vi "ImageCapture.vi"() -> ()   [LabVIEW 2021]
uses:
  <vilib>/userdefined/High Color/IMAQdx.ctl
  <vilib>/vision/driver/NI_Vision_Acquisition_Software.lvlib
panel:
  out "path":path
  out "error out 3":errorcluster
  in  "Ref":path
  in  "Snap?":bool
  out "error out 2":errorcluster
  out "error out":errorcluster
  out "Image":T1(plugin-control)
  in  "Camera Source":T2
  in  "stop":bool
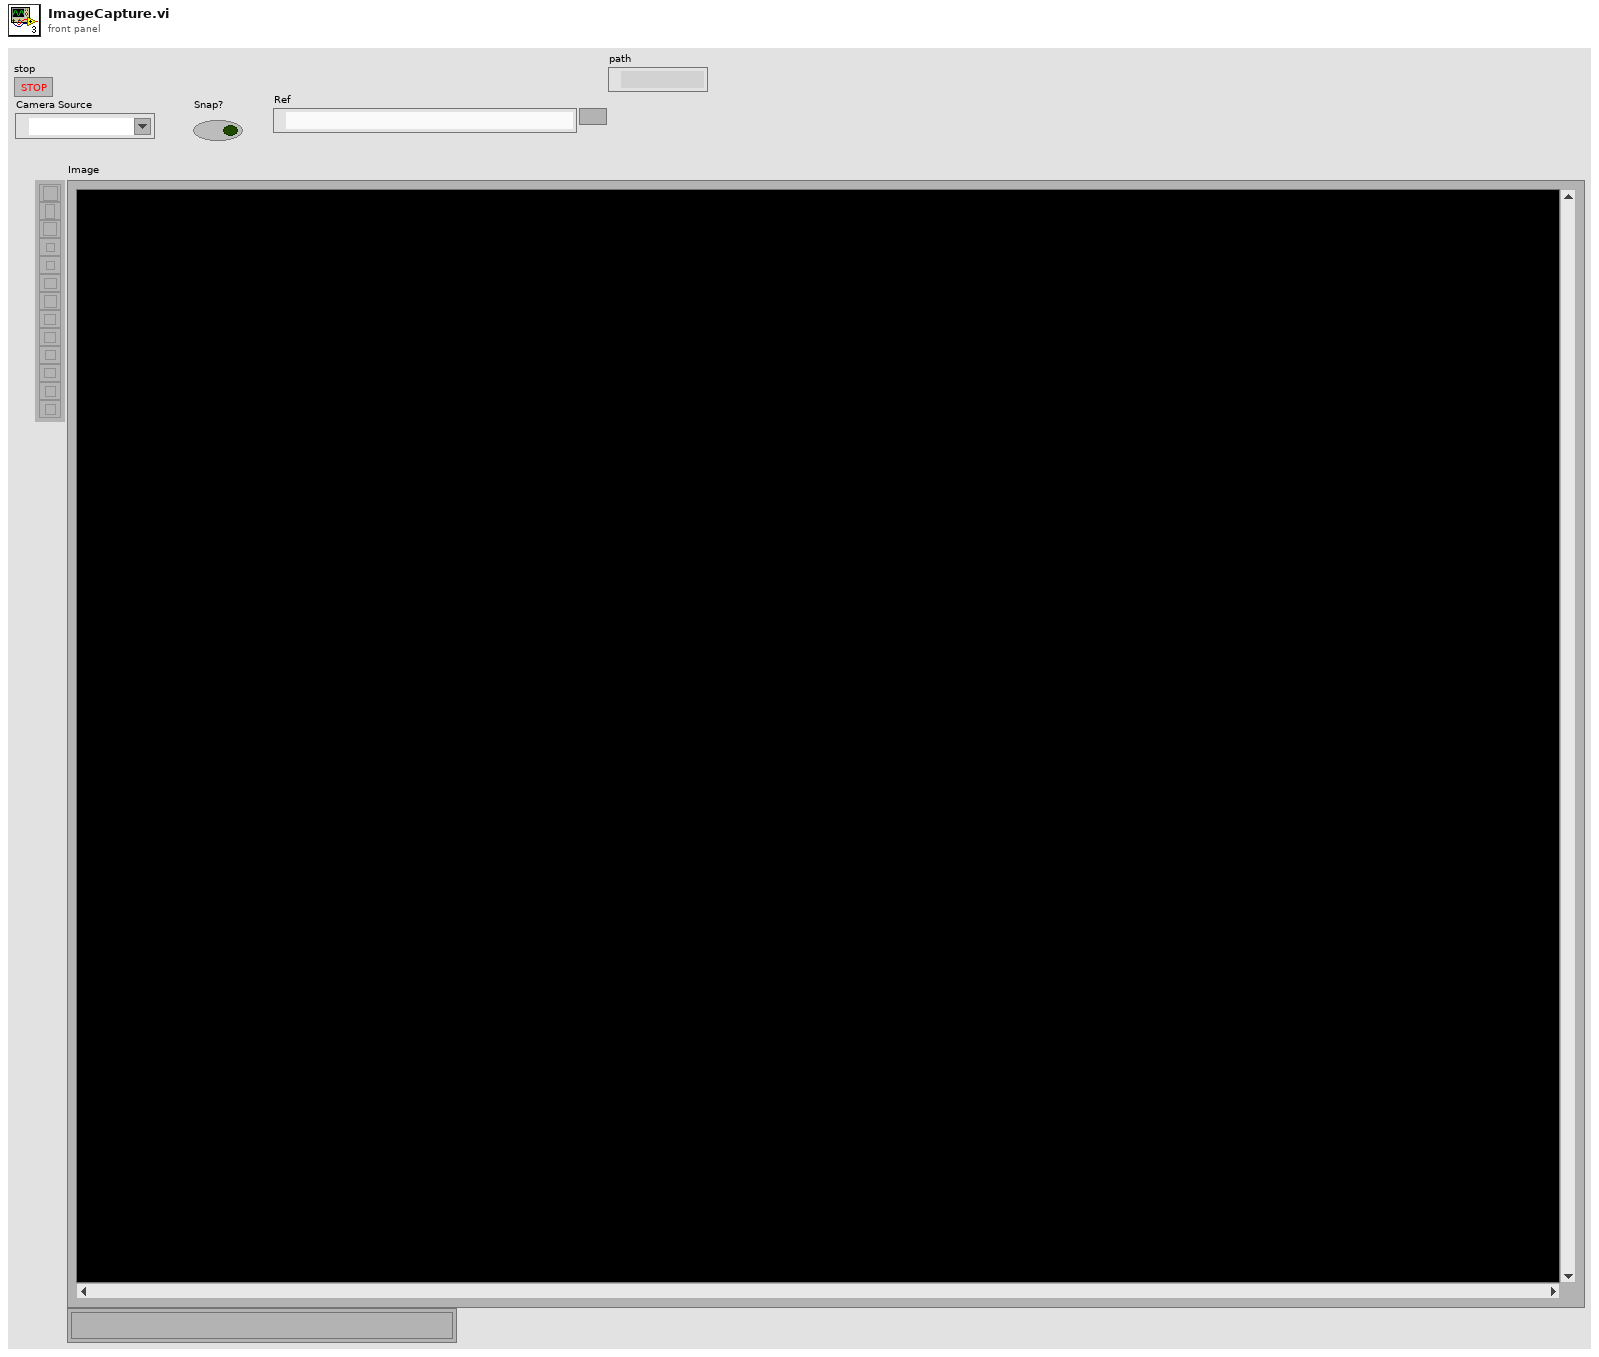
[diagram p1: front panel]
types:
  T1 = typedef "IMAQ Image.ctl" = refnum<image>
  T2 = typedef "IMAQdx.ctl" = refnum<k21>
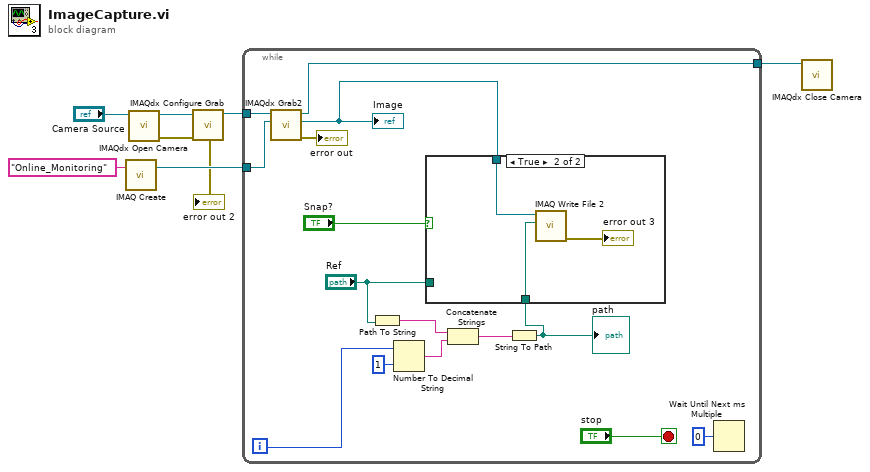
[diagram p0: block diagram]
diagram:
  n1 = call "IMAQ Create"("Image Name"="Online_Monitoring") -> ("New Image"=w4:T1)  [unwired: 4 in, 1 out]
  n2 = call <vilib>:"IMAQdx Open Camera.vi"("Session In"="Camera Source") -> ("error out"=w6:errorcluster, "Session Out"=w7:T2)  [unwired: 9 in]
  n3 = call <vilib>:"IMAQdx Configure Grab.vi"("error in"=w6, "Session In"=w7) -> ("error out"=→"error out 2":errorcluster, "Session Out"=w5:T2)  [unwired: 8 in]
  n4 = while {
    tunnel: w5 -> [w23]
    tunnel: w4 -> [w22]
    tunnel: [w20] -> w2
    i -> [w14]
    stop <- "stop" stop-if-true
    n5 = call <vilib>:"IMAQdx Grab2.vi"("Image In"=w22, "Session In"=w23) -> ("error out"=→"error out":errorcluster, "Image Out"=w16:T1, "Session Out"=w20:T2)  [unwired: 6 in, 1 out]
    "Image" <- w16
    n6 = Path To String(path="Ref") -> (string=w12:string)
    n7 = Number To Decimal String(number=w14, width (-)=i16 1) -> (decimal integer string=w11:string)
    n8 = Concatenate Strings(w12, w11) -> (w10:string)
    n9 = String To Path(string=w10) -> (path=w9:path)
    "path" <- w9
    n10 = case shown="True" "Snap?" {
      tunnel: w16 -> [_ w26]
      tunnel: "Ref" -> [_ _]
      tunnel: w9 -> [_ w24]
      frame False {
      }
      frame True {
        n11 = call-poly "IMAQ Write File 2"("File Path"=w24, "Image"=w26) -> ("error out"=→"error out 3":errorcluster)  [unwired: 8 in, 1 out]
      }
    }
    n12 = Wait Until Next ms Multiple(millisecond multiple=u32 0) -> ()  [unwired: 1 out]
  }
  n13 = call <vilib>:"IMAQdx Close Camera.vi"("Session In"=w2) -> ()  [unwired: 10 in, 1 out]
